vi "Launcher - UserInterface.vi"() -> ()   [LabVIEW 2021]
uses:
  Workers/UserInterface/UserInterface.lvclass
  C:/Program Files (x86)/National Instruments/LabVIEW 2021/vi.lib/addons/_Workers/Library/Classes/Worker/Worker.lvclass
  <vilib>/addons/_Workers/Debugger/Debug Client/Debug Client.lvlib
panel:
  out "error out":errorcluster
  in  "error in":errorcluster
  # "Launch Workers"
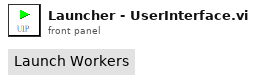
[diagram p1: front panel]
types:
  T1 = enum32{"Invalid", "Standard", "Closed", "Hidden", "Minimized", "Maximized"}
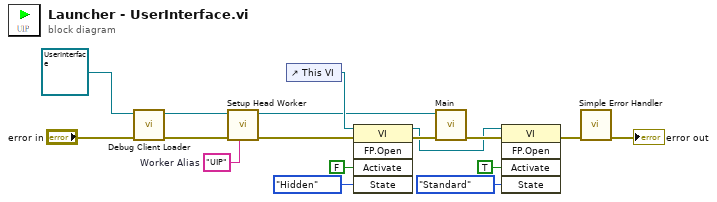
[diagram p0: block diagram]
diagram:
  w14 = "UIP"  # Worker Alias
  n1 = call <vilib>:"Debug Client Loader.vi"("error in (no error)"="error in", "Worker"=refnum<class "UserInterface.lvclass"> refnum ("Worker User Object")) -> ("error out"=w13:errorcluster, "Worker out"=w1:refnum<class "UserInterface.lvclass">)  [unwired: 8 in]
  n2 = call-dynamic "Setup Head Worker.vi"("Worker Alias"=w14, "error in"=w13, "Worker"=w1) -> ("error out"=w17:errorcluster, "Worker out"=w2:refnum<class "UserInterface.lvclass">)  [unwired: 7 in]
  n3 = control-ref of="This VI"() -> (w10:refnum<vi>)
  n4 = invoke class="VI" method="FP.Open"(reference=w10, error in=w17, "Activate"=FALSE ("Activate?"), "State"=T1."Hidden") -> (reference out=w3:refnum<vi>, error out=w11:errorcluster)  [unwired: 1 in, 3 out]
  n5 = call-dynamic "Main.vi"("error in"=w11, "UserInterface in"=w2) -> ("error out"=w5:errorcluster)  [unwired: 8 in, 1 out]
  n6 = invoke class="VI" method="FP.Open"(reference=w3, error in=w5, "Activate"=TRUE ("Activate?"), "State"=T1."Standard") -> (error out=w4:errorcluster)  [unwired: 1 in, 4 out]
  n7 = call <vilib>:"Simple Error Handler.vi"("error in (no error)"=w4) -> ("error out"=→"error out":errorcluster)  [unwired: 4 in, 4 out]
